vi "Drive.vi"(5 "Slow?":bool, 7 "SwitchDir":bool, 8 "Drive R":dbl, 11 "Drive L":dbl) -> ()   [LabVIEW 2017]
uses:
  <vilib>/Rock Robotics/WPI/SafetyOutput/WPI_SafetyOutputConfigMenu.ctl
panel:
  in  "Drive Reduction":dbl format="%#_13g"
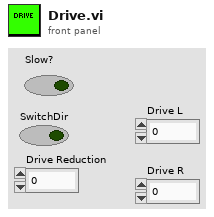
[diagram p1: front panel]
types:
  T1 = typedef "WPI_SafetyOutputConfigMenu.ctl" = enum16{"Enable", "Disable"}
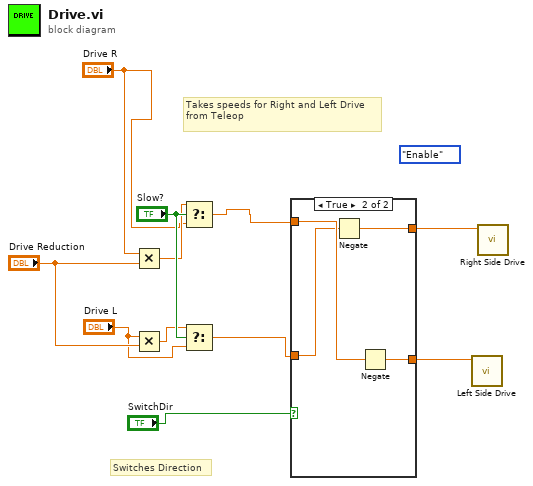
[diagram p0: block diagram]
diagram:
  (unwired) WPI_SafetyOutputConfigMenu."Enable" ("mode")
  # "Switches Direction"
  # "Takes speeds for Right and Left Drive\nfrom Teleop"
  n1 = Multiply(x="Drive R", y="Drive Reduction") -> (x*y=w7:dbl)
  n2 = Multiply(x="Drive L", y="Drive Reduction") -> (x*y=w5:dbl)
  n3 = Select(t=w7, s="Slow?", f="Drive R") -> (s? t:f=w3:dbl)
  n4 = Select(t=w5, s="Slow?", f="Drive L") -> (s? t:f=w10:dbl)
  n5 = case shown="True" "SwitchDir" {
    tunnel: [w13 w15] -> w2
    tunnel: w3 -> [w13 w17]
    tunnel: [w12 w14] -> w1
    tunnel: w10 -> [w12 w16]
    frame False {
    }
    frame True {
      n6 = Negate(x=w16) -> (-x=w15:dbl)
      n7 = Negate(x=w17) -> (-x=w14:dbl)
    }
  }
  n8 = call "Left Side Drive.vi"("Effort"=w1) -> ()  [unwired: 11 in]
  n9 = call "Right Side Drive.vi"("Effort"=w2) -> ()  [unwired: 11 in]
